vi "SigGen.vi"(8 "error in (no error)":errorcluster, 10 "SSTestInfoCluster":T1 {"Test InfoSS"."sample mode" items=["Finite Samples"=10178, "Continuous Samples"=10123, "Hardware Timed Single Point"=12522]}, 11 "E":dbl[][](array[numeric])) -> (0 "error out":errorcluster, 2 "DataSamples":dbl[][](array[numeric]), 3 "Generated waveforms":waveform(dbl)[](array[waveform]))   [LabVIEW 2014]
uses:
  TypeDefs/SSTestInfoCluster.ctl
  TypeDefs/SignalInfo.ctl
  TypeDefs/Test InfoSS.ctl
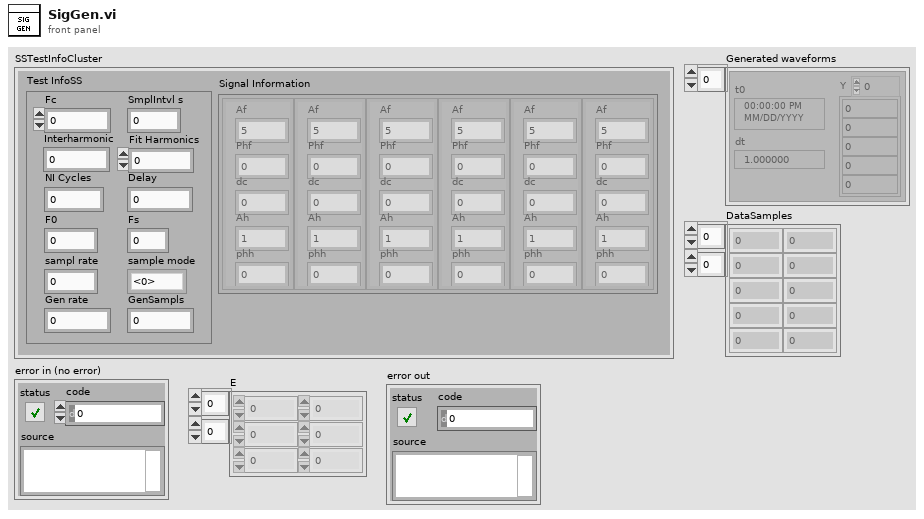
[diagram p1: front panel]
types:
  T1 = typedef "SSTestInfoCluster.ctl" = cluster{"Signal Information":T2, "Test InfoSS":T3}
  T2 = typedef "SignalInfo.ctl" = cluster{"Af":dbl, "Phf":dbl, "dc":dbl, "Ah":dbl, "phh":dbl}[]
  T3 = typedef "Test InfoSS.ctl" = cluster{"Fc":dbl, "Interharmonic":dbl, "Gen rate":dbl, "GenSampls":i32, "SmplIntvl s":dbl, "sampl rate":dbl, "sample mode":i32, "NI Cycles":dbl, "Delay":dbl, "Fit Harmonics":i32, "F0":dbl, "Fs":dbl}
  T4 = cluster{"Af":dbl, "Phf":dbl, "dc":dbl, "Ah":dbl, "phh":dbl}
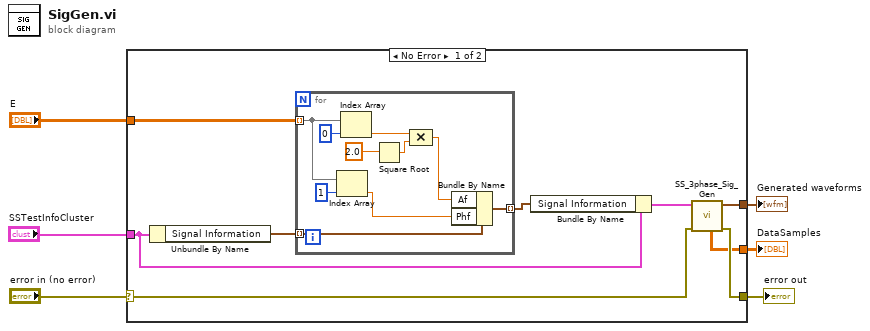
[diagram p0: block diagram]
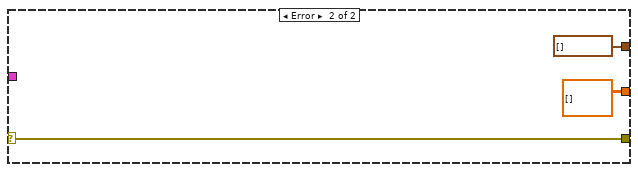
[diagram p2: hidden frame]
diagram:
  n1 = case shown="No Error" "error in (no error)" {
    selector: "error in (no error)" -> [w15 w28]
    tunnel: [w12 w28] -> w2
    tunnel: "SSTestInfoCluster" -> [w9 _]
    tunnel: "E" -> [w13 _]
    tunnel: [w8 waveform(dbl)[] [] ("Generated waveforms")] -> w5
    tunnel: [w7 dbl[][] [] ("DataSamples")] -> w6
    frame No Error {
      n2 = Unbundle By Name(w9) -> ("Signal Information"=w14:T2)
      n3 = for {
        tunnel: w14 -> [w25] mode=indexing
        tunnel: w13 -> [w24] mode=indexing
        tunnel: [w19] -> w10 mode=indexing
        n4 = Index Array(array=w24, index=1) -> (element=w20:dbl)
        n5 = Index Array(array=w24, index=0) -> (element=w21:dbl)
        n6 = Square Root(x=2.0) -> (sqrt(x)=w17:dbl)
        n7 = Compound Arithmetic op=MULTIPLY(w21, w17) -> (w18:dbl)
        n8 = Bundle By Name(cluster=w25, "Af"=w18, "Phf"=w20) -> (w19:T4)
      }
      n9 = Bundle By Name(cluster=w9, "Signal Information"=w10) -> (w11:T1)
      n10 = call "SS_3phase_Sig_Gen.vi"("error in (no error)"=w15, "SSTestInfoCluster"=w11) -> ("error out"=w12:errorcluster, "Generated waveforms"=w8:waveform(dbl)[], "DataSamples"=w7:dbl[][])  [unwired: 7 in]
    }
    frame Error {
    }
  }
  "DataSamples" <- w6
  "Generated waveforms" <- w5
  "error out" <- w2
